vi "Periodic Tasks.vi"(8 "error in":errorcluster) -> ()   [LabVIEW 2015]
doc: "This VI runs in parallel to other tasks. It can contain as many user-defined periodic loops as you need. These can carry out PID or other sorts of timed response."
uses:
  <vilib>/Rock Robotics/WPI/CAN/TalonSRX/WPI_CANTalonSRX_APIFeedbackSelect.ctl
  <vilib>/Rock Robotics/WPI/CAN/TalonSRX/WPI_CANTalonSRX_GlobalOps.ctl
  <vilib>/Rock Robotics/WPI/CAN/TalonSRX/WPI_CANTalonSRX_APIControlMode.ctl
  <vilib>/Rock Robotics/WPI/CAN/TalonSRX/WPI_CANTalonSRX_Params.ctl
  <vilib>/Rock Robotics/WPI/CAN/TalonSRX/WPI_CANTalonSRX_MotionProfileTrajectoryPt.ctl
  <vilib>/Rock Robotics/WPI/Utilities/WPI_GetSetVariantRefNum.vi
  <vilib>/Utility/file.llb/Read Delimited Spreadsheet (DBL).vi
panel:
  out "Mot Prof Active Position":dbl
  out "Mot Prof Active Velocity":dbl
  out "Mot Prof Output Enable":i32
  out "Mot Prof Count":i32
  out "Mot Prof NextID":i32
  out "Mot Prof Active Profile Slot Select":i32
  out "Mot Prof Buffer Is Full":bool
  out "Mot Prof Active Is Valid":bool
  out "Mot Prof Active Velocity Only":bool
  out "Mot Prof Active Is Last":bool
  out "Mot Prof  Has Under Run":bool
  out "Mot Prof  Is Under Run":bool
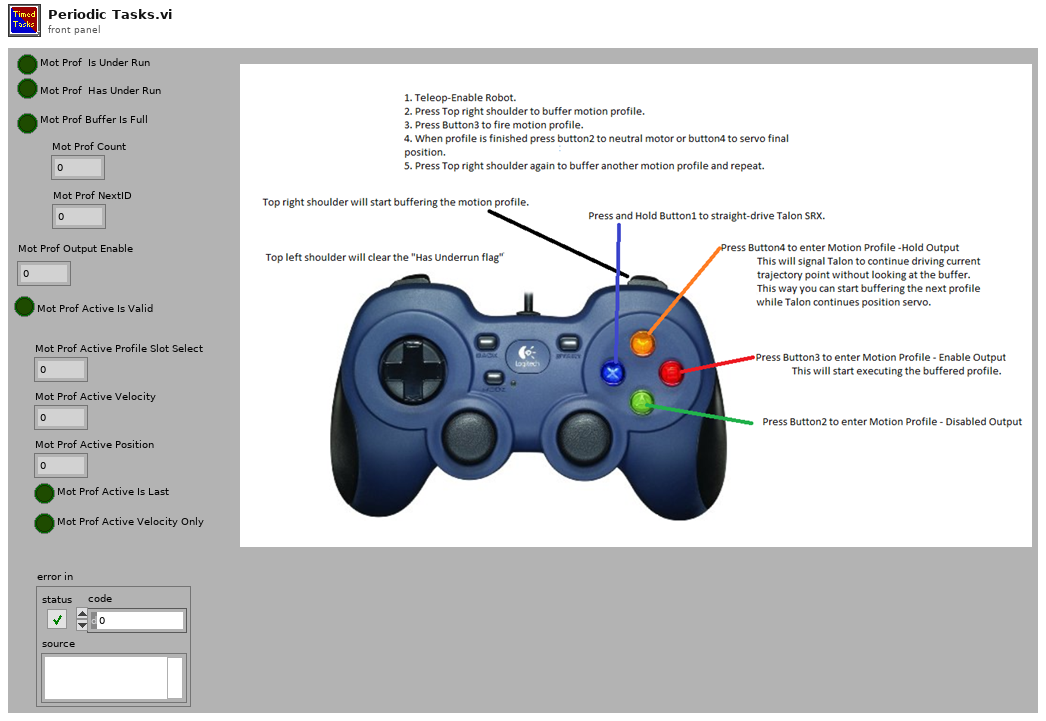
[diagram p1: front panel]
types:
  T1 = typedef "WPI_CANTalonSRX_GlobalOps.ctl" = enum16{"Read For Send", "Write After Receive General", "Write After Receive Feedback", "Write After Receive Encoder", "Write After Receive Ain", "Write Error", "Get All", "Set Output", "Set Mode", "Set Master ID", "Set Brake Mode", "Set Reverse Feedback Sensor", "Set Reverse Closed Loop Output", "Set Override Limits", "Set Forward Limit Enabled", "Set Reverse Limit Enabled", "Set Feedback Select", "Set Profile Select", "Set Throttle Ramp Rate", "Disable", "Set Enc Codes Per Rev", "Set Num Pot Turns", "Set Control Frame Rate", "Enable Legacy Control", "Write After Receive Pulse Width", "Set Enable Frame Rate", "Write After Receive Motion Profile", "Set Motion Profile Flow Control", "Set Motion Profile Control Frame Rate"}
  T2 = typedef "WPI_CANTalonSRX_APIFeedbackSelect.ctl" = enum16{"Digital Quadrature Encoder", "Analog Potentiometer", "Analog Encoder", "Count on Quad-A (Rising-Edge)", "Count on Quad-A (Falling-Edge)", "CTR Magnetic Enc (Absolute)", "CTR Magnetic Enc (Relative)", "Pulse Width"}
  T3 = typedef "WPI_MotorControlDeviceRef.ctl" = cluster{"DeviceStatus":errorcluster, "Type":T4, "PWM":cluster{"PWM Channel":T5, "DeadBand":T6}, "CAN":cluster{"Device Number":u8, "Control Mode":T7, "Semaphore":T8, "Max Vout":dbl, "TalonSRX Control Mode":T9}, "Invert":bool}
  T4 = typedef "WPI_MotorControlType.ctl" = enum16{"PWM", "CAN", "CANTalonSRX"}
  T5 = typedef "FPGA_DIOPWMChannel.ctl" = enum8{"PWM 0", "PWM 1", "PWM 2", "PWM 3", "PWM 4", "PWM 5", "PWM 6", "PWM 7", "PWM 8", "PWM 9", "PWM MXP 0", "PWM MXP 1", "PWM MXP 2", "PWM MXP 3", "PWM MXP 4", "PWM MXP 5", "PWM MXP 6", "PWM MXP 7", "PWM MXP 8", "PWM MXP 9", "Invalid"}
  T6 = typedef "WPI_PWMDeadband.ctl" = cluster{"Name":string, "maxPositivePwm":i32, "minPositivePwm":i32, "centerPwm":i32, "maxNegativePwm":i32, "minNegativePwm":i32, "angularRange":u16}
  T7 = typedef "WPI_CANJaguar_ControlMode.ctl" = enum8{"Percent VBus", "Current", "Speed", "Position", "Voltage"}
  T8 = typedef "Semaphore RefNum" = refnum<k1>
  T9 = typedef "WPI_CANTalonSRX_APIControlMode.ctl" = enum8{"Percent VBus", "Speed", "Position", "Slave", "Unchanged / Invalid", "Voltage Compensation", "Current", "Motion Profile"}
  T10 = typedef "WPI_JoystickDevRef.ctl" = cluster{"Device":T11}
  T11 = typedef "WPI_JoystickDeviceEnum.ctl" = enum16{"USB 0", "USB 1", "USB 2", "USB 3", "USB 4", "USB 5"}
  T12 = typedef "WPI_CANTalonSRX_MotionProfileTrajectoryPt.ctl" = cluster{"Duration Ms":u8, "Velocity":dbl, "Position":dbl, "Profile Slot Select":u8, "Is Last":bool, "Velocity Only":bool, "Zero Position":bool, "Compress Code":u8, "Same Velocity":i32, "Delta Position":i32, "Count":u8}
  T13 = typedef "WPI_CANTalonSRX_GlobalStatus.ctl" = cluster{"Applied Throttle":dbl, "Module Enabled":bool, "CAN Error":errorcluster, "Closed Loop Error":dbl, "Forward Limit Switch Closed":bool, "Reverse Limit Switch Closed":bool, "Sensor Position":dbl, "Sensor Velocity":dbl, "Current":dbl, "Sticky Fault - Over Temp":bool, "Sticky Fault - Under Voltage":bool, "Sticky Fault - Forward Limit":bool, "Sticky Fault - Reverse Limit":bool, "Sticky Fault - Forward Soft Limit":bool, "Sticky Fault - Reverse Soft Limit":bool, "Brake is Enabled":bool, "Encoder Position":dbl, "Encoder Velocity":dbl, "Encoder Index Count":dbl, "Encoder A Pin State":bool, "Encoder B Pin State":bool, "Encoder Index Pin State":bool, "Analog In":dbl, "Analog In Velocity":dbl, "Temperature (C)":dbl, "Battery Voltage":dbl, "Control 5 Is Supported":bool, "Current Profile Slot Select":dbl, "Pos Div 8":bool, "Vel Div 4":bool, "Pulse Width Position":i32, "Pulse Width Velocity":i32, "Pulse Width Rise To Rise (us)":i32, "Pulse Width Rise To Fall (us)":i32, "Mot Prof Active Is Under Run":bool, "Mot Prof Active Has Under Run":bool, "Mot Prof Active Is Last":bool, "Mot Prof Active Velocity Only":bool, "Mot Prof Active Is Valid":bool, "Mot Prof Buffer Is Full":bool, "Mot Prof Active Profile Slot Select":i32, "Mot Prof NextID":i32, "Mot Prof Count":i32, "Mot Prof Active Velocity":dbl, "Mot Prof Active Position":dbl, "Mot Prof Output Enable":i32}
  T14 = typedef "WPI_CANTalonSRX_Params.ctl" = u8
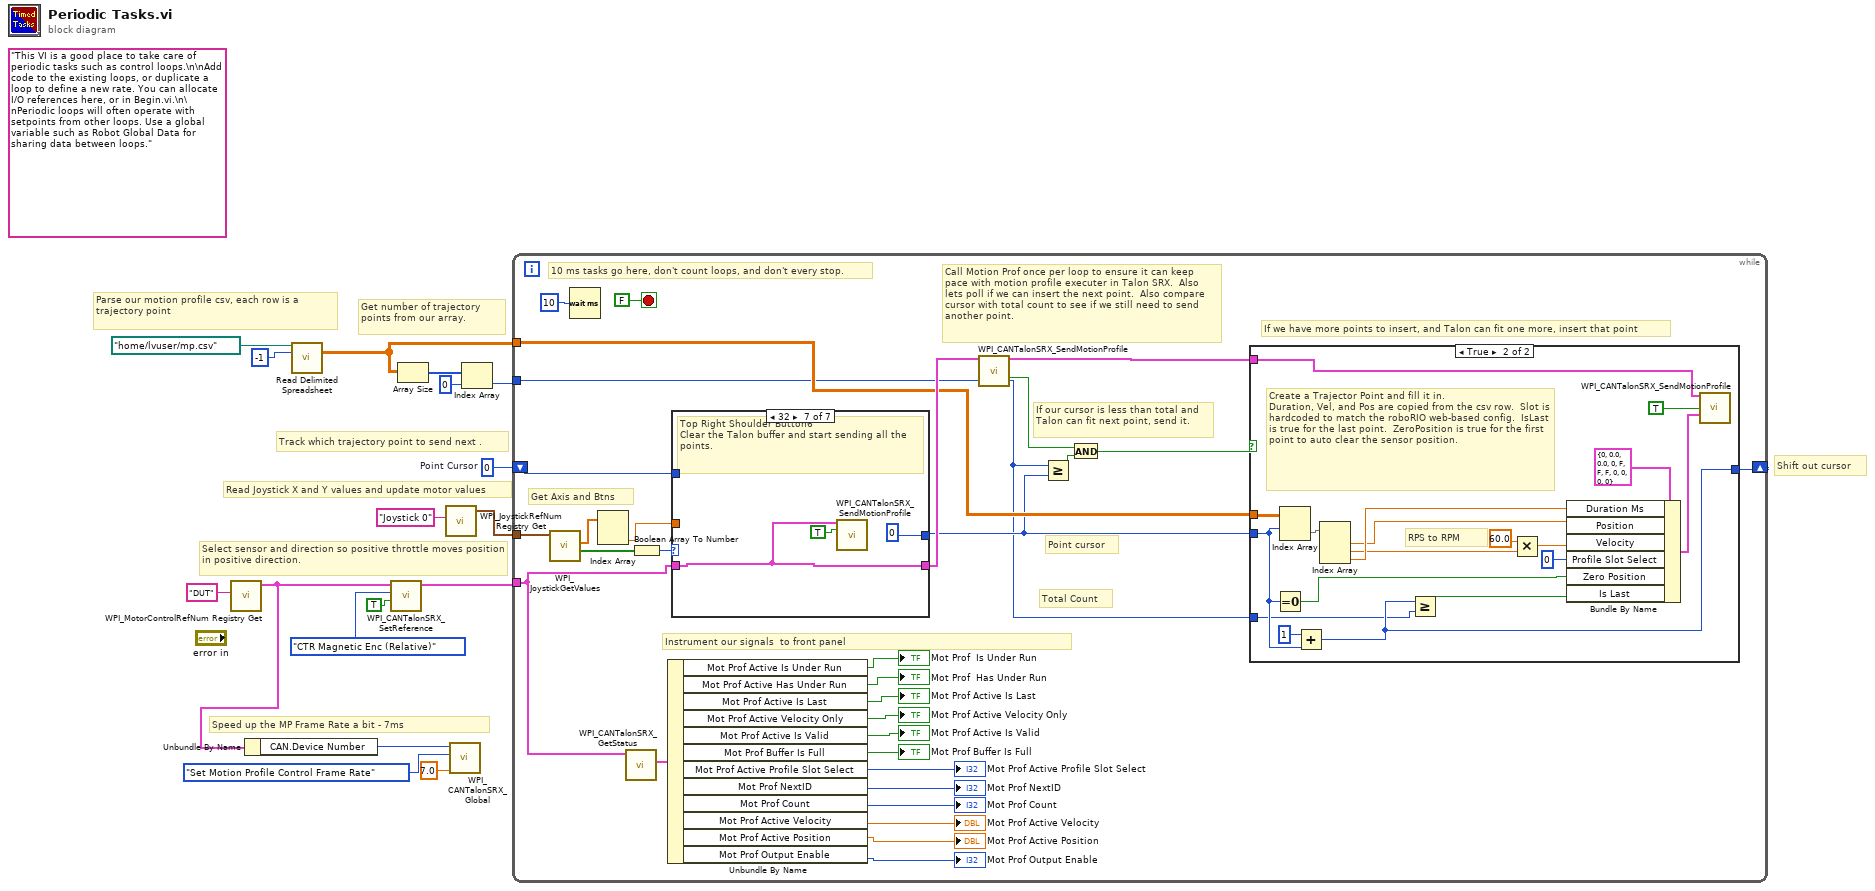
[diagram p0: block diagram]
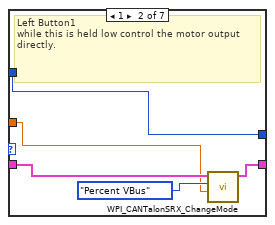
[diagram p4: hidden frame]
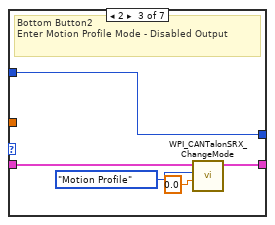
[diagram p5: hidden frame]
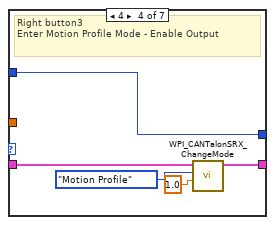
[diagram p6: hidden frame]
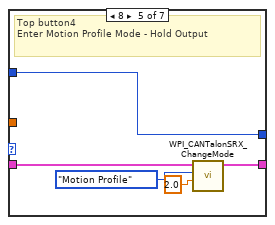
[diagram p7: hidden frame]
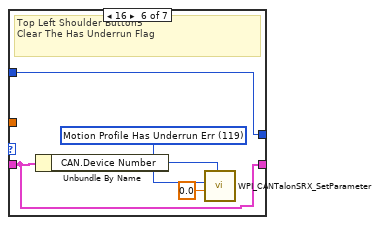
[diagram p8: hidden frame]
diagram:
  w12 = 0  # Point Cursor
  (unwired) "This VI is a good place to take care of periodic tasks such as control loops.\n\nAdd code to the existing loops, or duplicate a loop to define a new rate. You can allocate I/O references here, or in Begin.vi.\n\nPeriodic loops will often operate with setpoints from other loops. Use a global variable such as Robot Global Data for sharing data between loops."
  # "Select sensor and direction so positive throttle moves position in positive direction."
  # "Shift out cursor"
  # "Get number of trajectory points from our array."
  # "Track which trajectory point to send next ."
  # "Speed up the MP Frame Rate a bit - 7ms"
  # "Parse our motion profile csv, each row is a trajectory point"
  # "Read Joystick X and Y values and update motor values"
  n1 = call <vilib>:"WPI_MotorControlRefNum Registry Get.vi"("refnum name"="DUT") -> ("MotorControlDevRef"=w1:T3)  [unwired: 9 in, 1 out]
  n2 = Unbundle By Name(w1) -> ("CAN.Device Number"=w9:u8)
  n3 = call-poly <vilib>:"Read Delimited Spreadsheet.vi"("file path (dialog if empty)"=path "/home/lvuser/mp.csv" ("file path (use dialog)"), "number of rows (all:-1)"=-1) -> ("all rows"=w4:dbl[][])  [unwired: 8 in, 5 out]
  n4 = call <vilib>:"WPI_CANTalonSRX_SetReference.vi"("Reverse Feedback Sensor"=TRUE, "Feedback Reference"=WPI_CANTalonSRX_APIFeedbackSelect."CTR Magnetic Enc (Relative)", "CAN Talon SRX Ref"=w1) -> ("CAN Talon SRX Ref"=w2:T3)  [unwired: 7 in, 1 out]
  n5 = Array Size(array=w4) -> (size(s)=w5:i32[])
  n6 = call <vilib>:"WPI_JoystickRefNum Registry Get.vi"("refnum name"="Joystick 0") -> ("JoystickDevRef"=w15:T10)  [unwired: 1 in, 9 out]
  n7 = call <vilib>:"WPI_CANTalonSRX_Global.vi"("Set Number"=7.0, "Operation"=WPI_CANTalonSRX_GlobalOps."Set Motion Profile Control Frame Rate", "Device ID (0)"=w9) -> ()  [unwired: 6 in, 3 out]
  n8 = Index Array(array=w5, index=0) -> (element=w3:i32)
  n9 = while {
    tunnel: w15 -> [w43]
    tunnel: w4 -> [w41]
    shift-right: [w40] -> _
    shift-left: w12 -> [w25]
    tunnel: w3 -> [w22]
    tunnel: w2 -> [w18]
    stop <- FALSE stop-if-true
    # "Point cursor"
    # "Total Count"
    # "Get Axis and Btns"
    # "If our cursor is less than total and Talon can fit next point, send it."
    # "If we have more points to insert, and Talon can fit one more, insert that point"
    # "Call Motion Prof once per loop to ensure it can keep pace with motion profile executer in Talon SRX.  Also lets poll if we can insert the next point.  Also compare cursor with total count to see if we still need to send another point."
    # "Instrument our signals  to front panel"
    # "10 ms tasks go here, don't count loops, and don't every stop."
    n10 = call <vilib>:"WPI_JoystickGetValues.vi"("JoystickDevRef"=w43) -> ("Buttons"=w45:bool[], "Axes"=w46:dbl[])  [unwired: 6 in, 3 out]
    n11 = Wait (ms)(milliseconds to wait=u32 10) -> ()  [unwired: 1 out]
    n12 = Index Array(array=w46) -> (element #2=w39:dbl)  [unwired: 2 in, 1 out]
    n13 = call <vilib>:"WPI_CANTalonSRX_GetStatus.vi"("CAN Talon SRX Ref"=w18) -> ("Talon SRX Status"=w38:T13)  [unwired: 8 in, 2 out]
    n14 = Boolean Array To Number(Boolean array=w45) -> (number=w44:u32)
    n15 = Unbundle By Name(w38) -> ("Mot Prof Active Is Under Run"=→"Mot Prof  Is Under Run":bool, "Mot Prof Active Has Under Run"=→"Mot Prof  Has Under Run":bool, "Mot Prof Active Is Last"=→"Mot Prof Active Is Last":bool, "Mot Prof Active Velocity Only"=→"Mot Prof Active Velocity Only":bool, "Mot Prof Active Is Valid"=→"Mot Prof Active Is Valid":bool, "Mot Prof Buffer Is Full"=→"Mot Prof Buffer Is Full":bool, "Mot Prof Active Profile Slot Select"=→"Mot Prof Active Profile Slot Select":i32, "Mot Prof NextID"=→"Mot Prof NextID":i32, "Mot Prof Count"=→"Mot Prof Count":i32, "Mot Prof Active Velocity"=→"Mot Prof Active Velocity":dbl, "Mot Prof Active Position"=→"Mot Prof Active Position":dbl, "Mot Prof Output Enable"=→"Mot Prof Output Enable":i32)
    n16 = case shown="32" w44 {
      tunnel: w18 -> [w69 w73 w77 w82 w89 w91 w96]
      tunnel: [w69 w72 w76 w81 w86 w91 w96] -> w42
      tunnel: w39 -> [_ w71 _ _ _ _ _]
      tunnel: [w68 w70 w75 w80 w85 w90 0 ("Capacity")] -> w23
      tunnel: w25 -> [w68 w70 w75 w80 w85 w90 _]
      frame Default {
        # "No buttons we care about"
      }
      frame 1 {
        # "Left Button1\nwhile this is held low control the motor output directly."
        n17 = call <vilib>:"WPI_CANTalonSRX_ChangeMode.vi"("Output"=w71, "Control Mode"=WPI_CANTalonSRX_APIControlMode."Percent VBus", "CAN Talon SRX Ref"=w73) -> ("CAN Talon SRX Ref"=w72:T3)  [unwired: 7 in, 1 out]
      }
      frame 2 {
        # "Bottom Button2\nEnter Motion Profile Mode - Disabled Output"
        n18 = call <vilib>:"WPI_CANTalonSRX_ChangeMode.vi"("Output"=0.0, "Control Mode"=WPI_CANTalonSRX_APIControlMode."Motion Profile", "CAN Talon SRX Ref"=w77) -> ("CAN Talon SRX Ref"=w76:T3)  [unwired: 7 in, 1 out]
      }
      frame 4 {
        # "Right button3\nEnter Motion Profile Mode - Enable Output"
        n19 = call <vilib>:"WPI_CANTalonSRX_ChangeMode.vi"("Output"=1.0, "Control Mode"=WPI_CANTalonSRX_APIControlMode."Motion Profile", "CAN Talon SRX Ref"=w82) -> ("CAN Talon SRX Ref"=w81:T3)  [unwired: 7 in, 1 out]
      }
      frame 8 {
        # "Top button4\nEnter Motion Profile Mode - Hold Output"
        n20 = call <vilib>:"WPI_CANTalonSRX_ChangeMode.vi"("Output"=2.0, "Control Mode"=WPI_CANTalonSRX_APIControlMode."Motion Profile", "CAN Talon SRX Ref"=w89) -> ("CAN Talon SRX Ref"=w86:T3)  [unwired: 7 in, 1 out]
      }
      frame 16 {
        w94 = T14 119 items=["Slot 0 - P"=1, "Slot 0 - I"=2, "Slot 0 - D"=3, "Slot 0 - F"=4, "Slot 0 - I Zone"=5, "Slot 0 - Ramp Rate"=6, "Slot 1 - P"=11, "Slot 1 - I"=12, "Slot 1 - D"=13, "Slot 1 - F"=14, "Slot 1 - I Zone"=15, "Slot 1 - Ramp Rate"=16, "Soft Limit - Forward"=21, "Soft Limit - Reverse"=22, "Soft Limit - Forward Enable"=23, "Soft Limit - Reverse Enable"=24, "On Boot - Brake Mode"=31, "On Boot - Limit Normally Closed - Forward"=32, "On Boot - Limit Normally Closed - Reverse"=33, "On Boot - Limit Disabled - Forward"=34, "On Boot - Limit Disabled - Reverse"=35, "Fault - Over Temp"=41, "Fault - Under Voltage"=42, "Fault - Forward Limit"=43, "Fault - Reverse Limit"=44, "Fault - Hardware Failure"=45, "Fault - Forward Soft Limit"=46, "Fault - Reverse Soft Limit"=47, "Sticky Fault - Over Temp"=48, "Sticky Fault - Under Voltage"=49, "Sticky Fault - Forward Limit"=50, "Sticky Fault - Reverse Limit"=51, "Sticky Fault - Forward Soft Limit"=52, "Sticky Fault - Reverse Soft Limit"=53, "Applied Throttle"=61, "Closed-Loop Error"=62, "Select Feedback Device"=63, "Reverse Closed-Loop Output"=64, "Mode Select"=65, "Profile Slot Select"=66, "Ramp Throttle"=67, "Reverse Feedback Sensor"=68, "Limit Switch Enabled"=69, "Limit Switch Closed - Forward"=70, "Limit Switch Closed - Reverse"=71, "Sensor Position"=73, "Sensor Velocity"=74, "Current"=75, "Brake is Enabled"=76, "Encoder Position"=77, "Encoder Velocity"=78, "Encoder Index Rise Events"=79, "Encoder A Pin State"=80, "Encoder B Pin State"=81, "Encoder Index Pin State"=82, "Analog In with Overflow"=83, "Analog In Velocity"=84, "Temperature"=85, "Battery Voltage"=86, "Reset Count"=87, "Reset Flags"=88, "Firmware Version"=89, "Settings Changed"=90, "Quad Filter Enable"=91, "Ignore Disable Broadcast"=92, "I Accumulator"=93, "Status 1 Frame Rate Ms"=94, "Status 2 Frame Rate Ms"=95, "Status 3 Frame Rate Ms"=96, "Status 4 Frame Rate Ms"=97, "Status 6 Frame Rate Ms"=98, "Status 7 Frame Rate Ms"=99, "Enable Index Pin Clear Position"=100, "Peak Positive Output"=104, "Nominal Positive Output"=105, "Peak Negative Output"=106, "Nominal Negative Output"=107, "Quad Index Pin Polarity"=108, "Status 8 Frame Rate Ms"=109, "Allow Position Overflow"=110, "Slot 0 - Allowable Closed-Loop Error"=111, "Number Potentiometer Turns"=112, "Encoder Codes Per Rev"=113, "Pulse Width Decoded Position"=114, "Analog Position"=115, "Voltage Compensation Rate (V/s)"=116, "Slot 1 - Allowable Closed-Loop Error"=117, "Motion Profile Has Underrun Err"=119] ("Talon SRX Parameters")
        # "Top Left Shoulder Button5\nClear The Has Underrun Flag"
        n21 = Unbundle By Name(w91) -> ("CAN.Device Number"=w93:u8)
        n22 = call <vilib>:"WPI_CANTalonSRX_SetParameter.vi"("Value"=0.0, "Parameter"=w94, "Device ID (0)"=w93) -> ()  [unwired: 7 in, 2 out]
      }
      frame 32 {
        # "Top Right Shoulder Button6\nClear the Talon buffer and start sending all the points."
        n23 = call <vilib>:"WPI_CANTalonSRX_SendMotionProfile.vi"("CAN Talon SRX Ref"=w96, "Clear"=TRUE) -> ()  [unwired: 10 in, 4 out]
      }
    }
    n24 = call <vilib>:"WPI_CANTalonSRX_SendMotionProfile.vi"("CAN Talon SRX Ref"=w42) -> ("CAN Talon SRX Ref Out"=w21:T3, "Ready For Next"=w20:bool)  [unwired: 11 in, 2 out]
    n25 = Greater Or Equal?(x=w22, y=w23) -> (x >= y?=w19:bool)
    n26 = And(x=w20, y=w19) -> (x .and. y?=w24:bool)
    n27 = case shown="True" w24 {
      tunnel: w41 -> [_ w66]
      tunnel: [w49 w58] -> w40
      tunnel: w23 -> [w49 w59]
      tunnel: w22 -> [_ w50]
      tunnel: w21 -> [_ w55]
      frame False {
      }
      frame True {
        # "RPS to RPM"
        # "Create a Trajector Point and fill it in.\nDuration, Vel, and Pos are copied from the csv row.  Slot is hardcoded to match the roboRIO web-based config.  IsLast is true for the last point.  ZeroPosition is true for the first point to auto clear the sensor position."
        n28 = Equal To 0?(x=w59) -> (x = 0?=w51:bool)
        n29 = Index Array(array=w66, index (row)=w59) -> (element=w62:dbl[])  [unwired: 1 in]
        n30 = Add(x=u32 1, y=w59) -> (x+y=w58:u32)
        n31 = Index Array(array=w62) -> (element #1=w54:dbl, element #2=w56:dbl, element #3=w61:dbl)  [unwired: 3 in]
        n32 = Greater Or Equal?(x=w58, y=w50) -> (x >= y?=w52:bool)
        n33 = Multiply(x=60.0, y=w56) -> (x*y=w53:dbl)
        n34 = Bundle By Name(cluster=T12 {"Duration Ms"=0, "Velocity"=0.0, "Position"=0.0, "Profile Slot Select"=0, "Is Last"=FALSE, "Velocity Only"=FALSE, "Zero Position"=FALSE, "Compress Code"=0, "Same Velocity"=0, "Delta Position"=0, "Count"=0} ("New Point"), "Duration Ms"=w61, "Position"=w54, "Velocity"=w53, "Profile Slot Select"=u8 0, "Zero Position"=w51, "Is Last"=w52) -> (w63:T12)
        n35 = call <vilib>:"WPI_CANTalonSRX_SendMotionProfile.vi"("CAN Talon SRX Ref"=w55, "Push"=TRUE, "New Point"=w63) -> ()  [unwired: 9 in, 4 out]
      }
    }
  }
